vi "Check.vi"(0 "reference in":refnum<class "Cylinder.lvclass">, 5 "error in (no error)":errorcluster) -> (14 "reference out":refnum<class "Cylinder.lvclass">, 19 "error out":errorcluster)   [LabVIEW 2013, in "Cylinder.lvclass"]
uses:
  Cylinder.lvclass
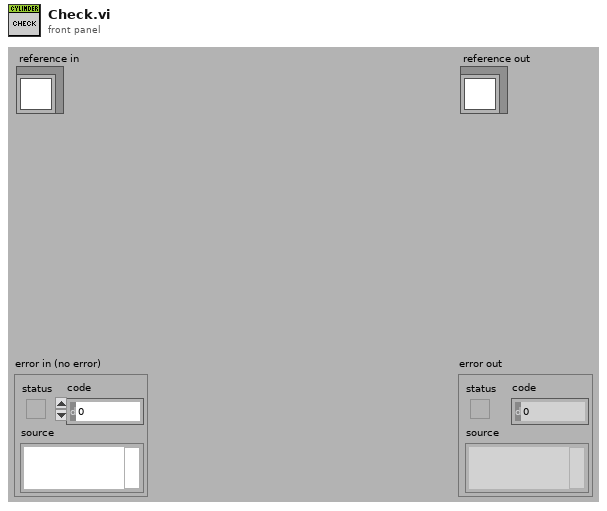
[diagram p1: front panel]
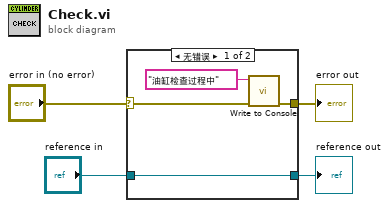
[diagram p0: block diagram]
diagram:
  n1 = case shown="无错误" "error in (no error)" {
    selector: "error in (no error)" -> [w7 w10]
    tunnel: [w6 w10] -> w3
    tunnel: [w5 w9] -> w1
    tunnel: "reference in" -> [w5 w9]
    frame No Error {
      n2 = call "Write to Console.vi"("error in (no error)"=w7, "Input"="油缸检查过程中") -> ("error out"=w6:errorcluster)  [unwired: 9 in]
    }
    frame Error {
    }
  }
  "error out" <- w3
  "reference out" <- w1
